vi "Take_Data.vi"(1 "Samples Before Frequency Change":i32[](array[numeric]), 2 "Samples Before Measuring":i32[](array[numeric]), 3 "Current Frequency Index":i32, 4 "Current Sample":i32) -> (0 "Take Data":bool)   [LabVIEW 2017]
doc: "If the current sample is greater than the last sample to be ignored and less than or equal to the last sample taken before changing frequencies for the current frequency, take data.\n\nInputs:\n\n- Current Sample: The current sample being measured of the excited system. \n NOTE: Since we must excite the system before recording data, this will be the number of iterations the loop containing this function has run minus one.\n\n- Samples Before Measuring: A list of the last sample ignored at each frequency. Measuring should begin following this sample.\n\n- Samples Before Frequency Change: A list of the indices of the last sample taken at a particular frequency before the frequency changes. The following sample, the excitaton frequency changes. \n\n- Current Frequency Index: The index of the current frequency used to generate the sine wave which excited the system. This index determines which sample before measuring and sample before frequency change the current sample should be between for data to be collected.\n\nOutput:\n\n- Take Data: TRUE = good to take data / FALSE = do not take data"
panel:
  # "Take_Data"
  # "Current State"
  # "Points To Take Data Between"
  # "Measuring"
  # "Frequency Change"
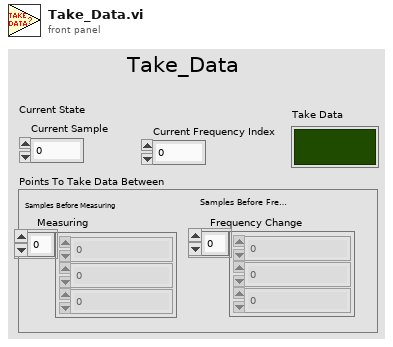
[diagram p1: front panel]
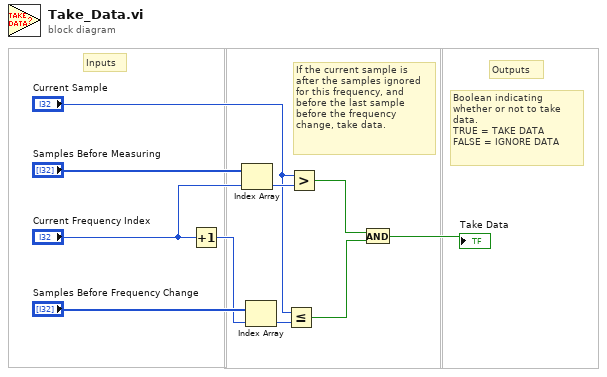
[diagram p0: block diagram]
diagram:
  # "Boolean indicating whether or not to take data.\nTRUE = TAKE DATA\nFALSE = IGNORE DATA"
  # "Outputs"
  # "If the current sample is after the samples ignored for this frequency, and before the last sample before the frequency change, take data."
  # "Inputs"
  n1 = Increment(x="Current Frequency Index") -> (x+1=w7:i32)
  n2 = Index Array(array="Samples Before Measuring", index="Current Frequency Index") -> (element=w6:i32)
  n3 = Index Array(array="Samples Before Frequency Change", index=w7) -> (element=w5:i32)
  n4 = Less Or Equal?(x="Current Sample", y=w5) -> (x <= y?=w2:bool)
  n5 = Greater?(x="Current Sample", y=w6) -> (0:w3:bool)
  n6 = And(x=w3, y=w2) -> (x .and. y?=→"Take Data":bool)
